vi "Initialize Rx Channels and Label Buffers.vi"(8 "error in":errorcluster, 10 "module handle":u8, 11 "Rx Channels in":T1[](array[typedef]) {"labels settings for RT"."Label Timestamp Channel Data Reference" format="%.0x"; "labels settings for RT"."Word Initial Raw Value" format="%032.0f"; "labels settings for RT"."Label Disable/Trigger Channel Reference" format="%.0x"; "labels settings for RT"."parameter driver data"."Tx parameter refs" format="%.0x"; "labels settings for RT"."SDI" format="%02b"; "labels settings for RT"."label" format="%.0o"}) -> (0 "error out":errorcluster, 3 "Rx Channels out":T1[](array[typedef]) {"labels settings for RT"."Label Timestamp Channel Data Reference" format="%.0x"; "labels settings for RT"."Word Initial Raw Value" format="%032.0f"; "labels settings for RT"."Label Disable/Trigger Channel Reference" format="%.0x"; "labels settings for RT"."parameter driver data"."Tx parameter refs" format="%.0x"; "labels settings for RT"."SDI" format="%02b"; "labels settings for RT"."label" format="%.0o"})   [LabVIEW 2020, in "AIM ARINC 429 Hardware API.lvlib"]
uses:
  AIM ARINC 429 Hardware API.lvlib
  <instrlib>/AIM GmbH/ARINC-429/AIM429LV.lvlib
  <instrlib>/AIM GmbH/ARINC-429/Session/controls/api429_rx_label_setup.ctl
  <instrlib>/AIM GmbH/ARINC-429/Session/Session.lvclass
  Shared/Label.ctl
  <vilib>/NI/NI VeriStand Encoding and Decoding/Encoding.ctl
  <vilib>/NI/NI VeriStand Encoding and Decoding/Encoding and Decoding.lvlib
  Shared/Parameter Definition.ctl
  <vilib>/NI VeriStand/Custom Device API/Custom Device Item Ref.ctl
  <vilib>/NI VeriStand/Custom Device API/Custom Device API.lvlib
  Shared/RT Parameters.ctl
  Shared/Transfer Type.ctl
  <vilib>/NI VeriStand/Custom Device API/Data Reference.ctl
  Shared/RT Label Settings.ctl
  Shared/RT Hardware Channel Settings.ctl
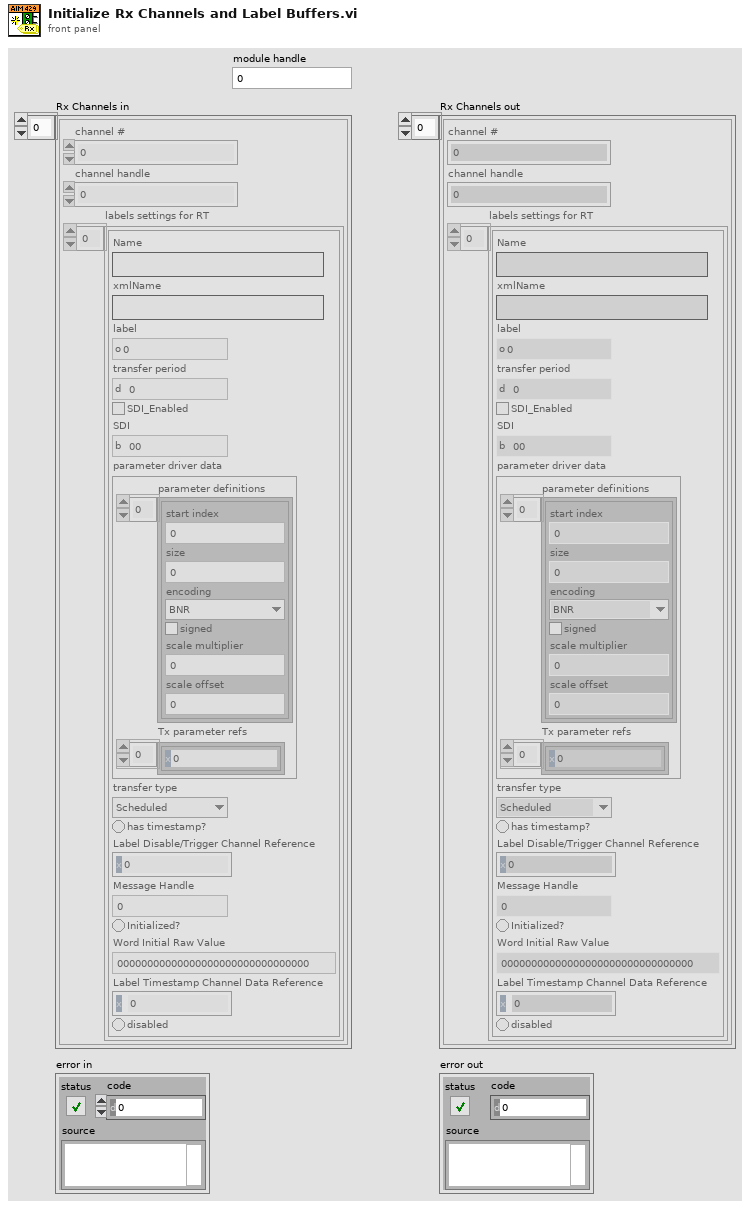
[diagram p1: front panel]
types:
  T1 = typedef "RT Hardware Channel Settings.ctl" = cluster{"channel #":u16, "channel handle":u64, "labels settings for RT":T2[]}
  T2 = typedef "RT Label Settings.ctl" = cluster{"Name":string, "xmlName":string, "label":T3, "transfer period":u32, "SDI_Enabled":bool, "SDI":u8, "parameter driver data":T4, "transfer type":T8, "has timestamp?":bool, "Label Disable/Trigger Channel Reference":T7, "Message Handle":u64, "Initialized?":bool, "Word Initial Raw Value":u32, "Label Timestamp Channel Data Reference":T9, "disabled":bool}
  T3 = typedef "Label.ctl" = u8
  T4 = typedef "RT Parameters.ctl" = cluster{"parameter definitions":T5[], "Tx parameter refs":T7[]}
  T5 = typedef "Parameter Definition.ctl" = cluster{"start index":i32, "size":i32, "encoding":T6, "signed":bool, "scale multiplier":dbl, "scale offset":dbl}
  T6 = typedef "Encoding and Decoding.lvlib/Encoding.ctl" = enum16{"BNR", "BCD", "Discrete"}
  T7 = typedef "Custom Device API.lvlib/Custom Device Item Ref.ctl" = u64
  T8 = typedef "Transfer Type.ctl" = enum16{"Scheduled", "Acyclic", "Block", "Strobe"}
  T9 = typedef "Custom Device API.lvlib/Data Reference.ctl" = i32
  T10 = typedef "AIM429LV.lvlib/Session.lvclass/api429_rx_label_setup.ctl" = cluster{"label number":u32, "sdi":u32, "label control flag":u32, "interrupt control flag":u32, "interrupt index":u32, "buffer size":u32}
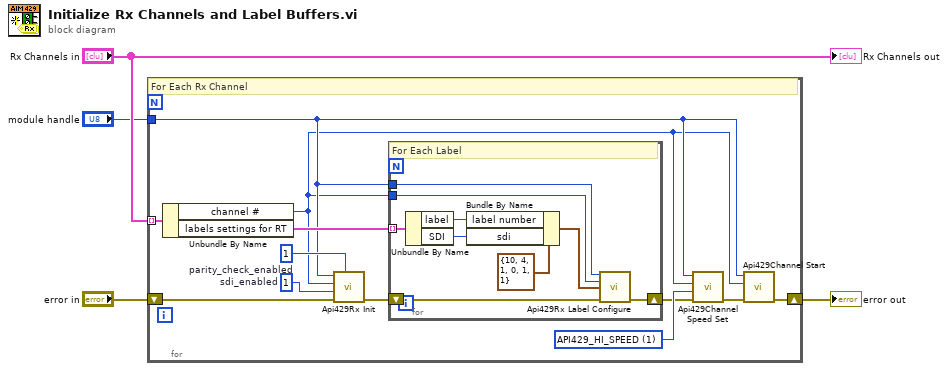
[diagram p0: block diagram]
diagram:
  n1 = for {
    tunnel: "Rx Channels in" -> [w16] mode=indexing
    shift-right: [w10] -> w2
    shift-left: "error in" -> [w15]
    tunnel: "module handle" -> [w6]
    w11 = u32 1 items=["API429_LO_SPEED", "API429_HI_SPEED"] ("speed")
    w13 = u8 1  # sdi_enabled
    w14 = u8 1  # parity_check_enabled
    # "For Each Rx Channel"
    n2 = Unbundle By Name(w16) -> ("channel #"=w5:u16, "labels settings for RT"=w12:T2[])
    n3 = call <instrlib>:"Api429Rx Init.vi"("parity_check_enabled"=w14, "error in (no error)"=w15, "sdi_enabled"=w13, "b_Chn"=w5, "board_handle"=w6) -> ("error out"=w7:errorcluster)  [unwired: 6 in]
    n4 = for {
      shift-right: [w17] -> w8
      shift-left: w7 -> [w24]
      tunnel: w6 -> [w25]
      tunnel: w5 -> [w23]
      tunnel: w12 -> [w22] mode=indexing
      # "For Each Label"
      n5 = Unbundle By Name(w22) -> ("label"=w20:T3, "SDI"=w19:u8)
      n6 = Bundle By Name(cluster=T10 {"label number"=10, "sdi"=4, "label control flag"=1, "interrupt control flag"=0, "interrupt index"=1, "buffer size"=1} ("rx parameters"), "label number"=w20, "sdi"=w19) -> (w18:T10)
      n7 = call <instrlib>:"Api429Rx Label Configure.vi"("board_handle"=w25, "b_Chn"=w23, "label_setup"=w18, "error in (no error)"=w24) -> ("error out"=w17:errorcluster)  [unwired: 9 in, 2 out]
    }
    n8 = call <instrlib>:"Api429Channel Speed Set.vi"("error in (no error)"=w8, "speed"=w11, "b_Chn"=w5, "board_handle"=w6) -> ("error out"=w9:errorcluster)  [unwired: 7 in]
    n9 = call <instrlib>:"Api429Channel Start.vi"("error in (no error)"=w9, "channel_id"=w5, "board_handle"=w6) -> ("error out"=w10:errorcluster)  [unwired: 8 in]
  }
  "error out" <- w2
  "Rx Channels out" <- "Rx Channels in"
